vi "fgv_ctrl-ref_old2.vi"(7 "cmd":enum16{"read", "write"}(ring), 11 "ref in":T1) -> (3 "ref out":T1)   [LabVIEW 2019]
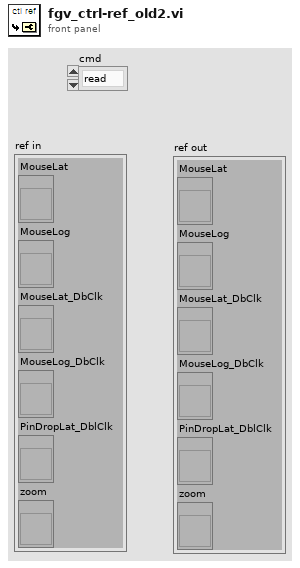
[diagram p1: front panel]
types:
  T1 = cluster{"MouseLat":refnum<vi>, "MouseLog":refnum<vi>, "MouseLat_DbClk":refnum<vi>, "MouseLog_DbClk":refnum<vi>, "PinDropLat_DblClk":refnum<vi>, "zoom":refnum<vi>}
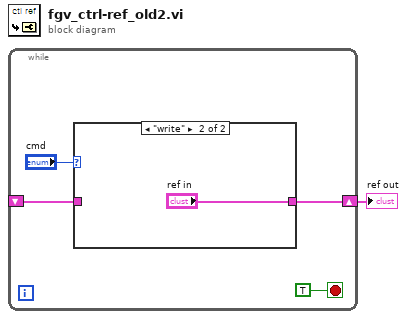
[diagram p0: block diagram]
diagram:
  n1 = while {
    shift-right: [w3] -> w1
    shift-left: _ -> [w2]
    stop <- TRUE stop-if-true
    n2 = case shown="\"write\"" "cmd" {
      tunnel: [w6 "ref in"] -> w3
      tunnel: w2 -> [w6 _]
      frame "read", Default {
      }
      frame "write" {
      }
    }
  }
  "ref out" <- w1
